vi "vectorstore_polymorphic.vi"   [LabVIEW 2020]
uses:
  vector_qdrant/vector_qdrant.lvclass
  vector_weviate/vector_weviate.lvclass
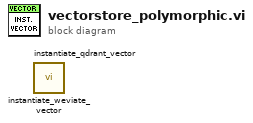
[diagram p0: block diagram]
diagram:
  n1 = call "instantiate_weviate_vector.vi"() -> ()  [unwired: 14 in, 2 out]
  n2 = call "instantiate_qdrant_vector.vi"() -> ()  [unwired: 14 in, 2 out]
